vi "Part 2.vi"() -> ()   [LabVIEW 2020]
uses:
  <vilib>/Utility/file.llb/Read Delimited Spreadsheet (string).vi
panel:
  in  "Selection":enum16{"Name", "Country of Birth", "Age"}(ring)
  out "Histogram Graph":cluster{i32[], i32[]}(graph)
  out "sum":i32
  out "Array":string[](array[string])
  out "Map":map{string, i32}(c390)
  in  "Path":path
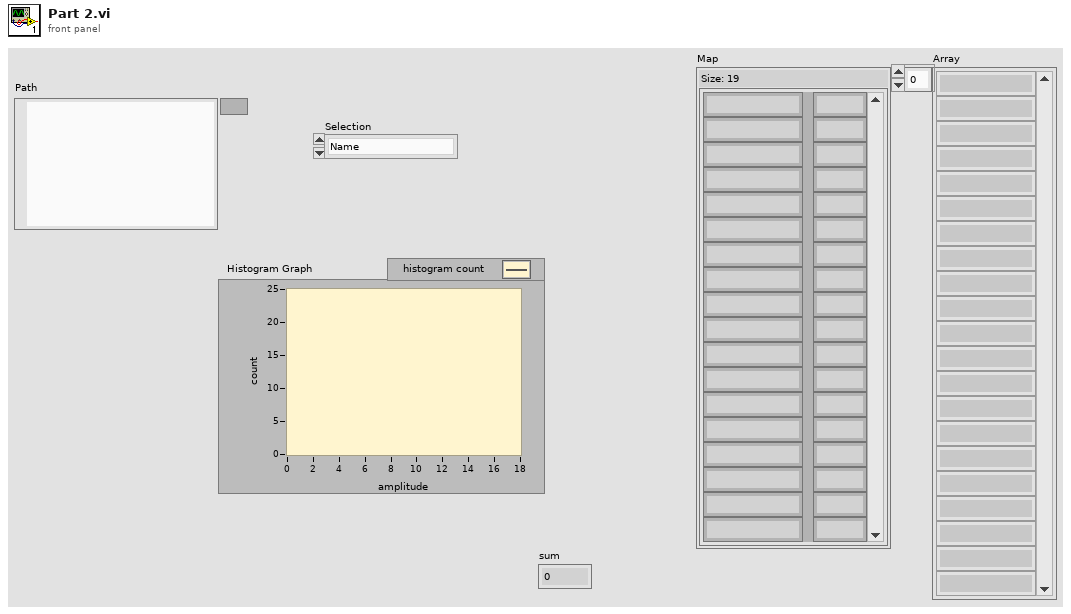
[diagram p1: front panel]
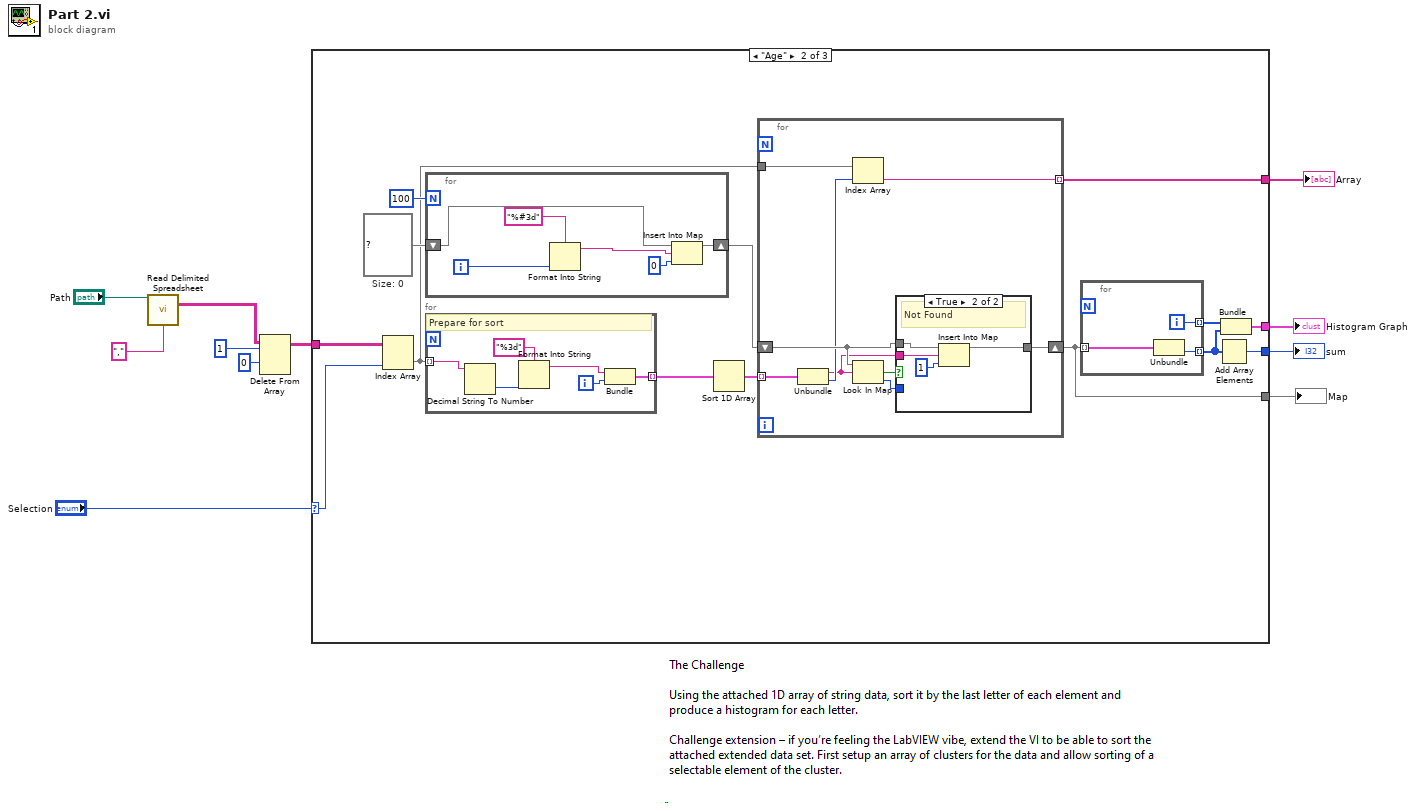
[diagram p0: block diagram]
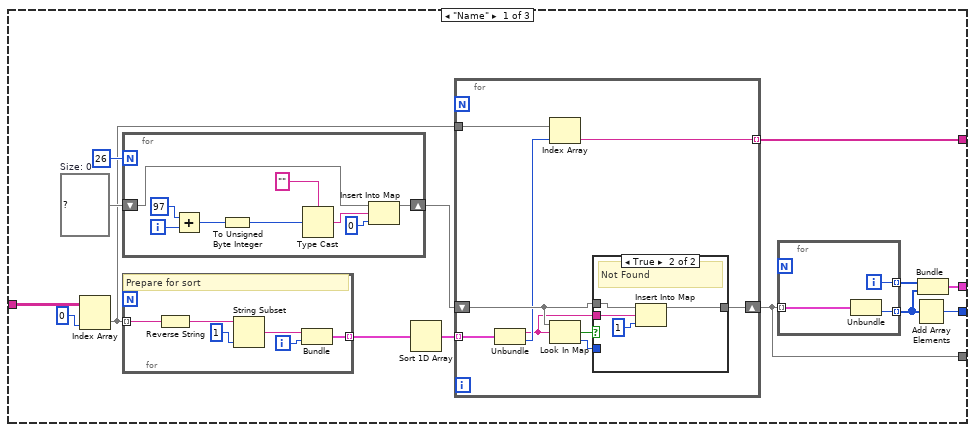
[diagram p2: hidden frame]
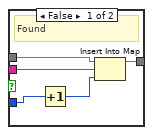
[diagram p3: hidden frame]
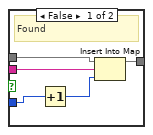
[diagram p4: hidden frame]
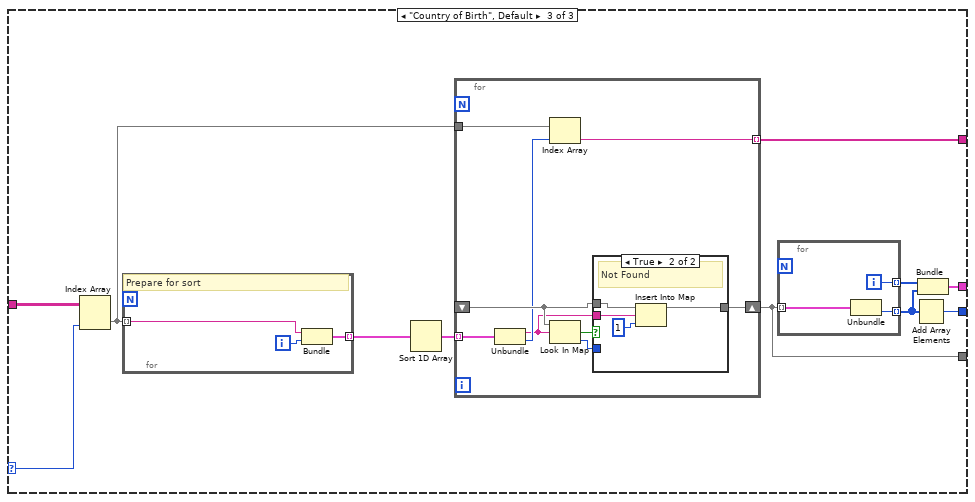
[diagram p5: hidden frame]
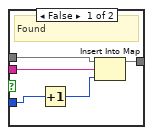
[diagram p6: hidden frame]
diagram:
  n1 = call-poly <vilib>:"Read Delimited Spreadsheet.vi"("file path (dialog if empty)"="Path", "delimiter (\\t)"="," ("delimiter (\\t)")) -> ("all rows"=w4:string[][])  [unwired: 8 in, 5 out]
  n2 = Delete From Array(array=w4, length=1, index (row)=0) -> (array with subset deleted=w3:string[][])  [unwired: 1 in, 1 out]
  n3 = case shown="\"Age\"" "Selection" {
    selector: "Selection" -> [_ w62 w109]
    tunnel: w3 -> [w25 w75 w119]
    tunnel: [w17 w68 w115] -> w9
    tunnel: [w16 w67 w114] -> w8
    tunnel: [w15 w66 w113] -> w7
    tunnel: [w14 w65 w112] -> w6
    frame "Name" {
      w22 = map{string, i32} {}  # Size: 0
      n4 = Index Array(array=w25, index (col)=0 ("disabled index (col)")) -> (element=w18:string[])  [unwired: 1 in]
      n5 = for {
        N: 26 -> [_]
        shift-right: [w50] -> w19
        shift-left: w22 -> [w51]
        i -> [w54]
        n6 = Add(x=97, y=w54) -> (x+y=w53:i32)
        n7 = To Unsigned Byte Integer(number=w53) -> (unsigned 8bit integer=w47:u8)
        n8 = Type Cast(type="", x=w47) -> (*(type *) &x=w49:string)
        n9 = Insert Into Map(map in=w51, key=w49, value=0) -> (map out=w50:map{string, i32})  [unwired: 2 out]
      }
      n10 = for {
        tunnel: w18 -> [w61] mode=indexing
        tunnel: [w56] -> w23 mode=indexing
        i -> [w57]
        # "Prepare for sort"
        n11 = Reverse String(1:w61) -> (0:w60:string)
        n12 = String Subset(string=w60, length (rest)=1 ("length (rest)")) -> (substring=w58:string)  [unwired: 1 in]
        n13 = Bundle(w58, w57) -> (w56:cluster{string, i32})  [unwired: 1 in]
      }
      n14 = Sort 1D Array(array=w23) -> (sorted array=w20:cluster{string, i32}[])
      n15 = for {
        tunnel: w20 -> [w37] mode=indexing
        shift-right: [w32] -> w16
        shift-left: w19 -> [w33]
        tunnel: w18 -> [w36]
        tunnel: [w35] -> w17 mode=indexing
        n16 = Unbundle(w37) -> (w30:string, w31:i32)
        n17 = Index Array(array=w36, index=w31) -> (element=w35:string)
        n18 = Look In Map(map=w33, key=w30) -> (key not found?=w34:bool, value=w29:i32)  [unwired: 1 in]
        n19 = case shown="True" w34 {
          tunnel: w33 -> [w42 w45]
          tunnel: [w41 w46] -> w32
          tunnel: w30 -> [w40 w44]
          tunnel: w29 -> [w39 _]
          frame False {
            # "Found"
            n20 = Increment(x=w39) -> (x+1=w38:i32)
            n21 = Insert Into Map(map in=w42, key=w40, value=w38) -> (map out=w41:map{string, i32})  [unwired: 2 out]
          }
          frame True {
            # "Not Found"
            n22 = Insert Into Map(map in=w45, key=w44, value=1) -> (map out=w46:map{string, i32})  [unwired: 2 out]
          }
        }
      }
      n23 = for {
        tunnel: w16 -> [w28] mode=indexing
        tunnel: [w27] -> w13 mode=indexing
        tunnel: [w26] -> w12 mode=indexing
        i -> [w26]
        n24 = Unbundle(w28) -> (w27:i32)  [unwired: 1 out]
      }
      n25 = Add Array Elements(numeric array=w13) -> (sum=w15:i32)
      n26 = Bundle(w12, w13) -> (w14:cluster{i32[], i32[]})  [unwired: 1 in]
    }
    frame "Age" {
      w73 = map{string, i32} {}  # Size: 0
      n27 = Index Array(array=w75, index (col)=w62) -> (element=w69:string[])  [unwired: 1 in]
      n28 = for {
        N: 100 -> [_]
        shift-right: [w101] -> w70
        shift-left: w73 -> [w102]
        i -> [w98]
        n29 = Format Into String(format string="%#3d", w98) -> (resulting string=w97:string)  [unwired: 2 in, 1 out]
        n30 = Insert Into Map(map in=w102, key=w97, value=0) -> (map out=w101:map{string, i32})  [unwired: 2 out]
      }
      n31 = for {
        tunnel: w69 -> [w104] mode=indexing
        tunnel: [w107] -> w74 mode=indexing
        i -> [w108]
        # "Prepare for sort"
        n32 = Decimal String To Number(string=w104) -> (number=w105:i32)  [unwired: 2 in, 1 out]
        n33 = Format Into String(format string="%3d", w105) -> (resulting string=w103:string)  [unwired: 2 in, 1 out]
        n34 = Bundle(w103, w108) -> (w107:cluster{string, i32})  [unwired: 1 in]
      }
      n35 = Sort 1D Array(array=w74) -> (sorted array=w71:cluster{string, i32}[])
      n36 = for {
        tunnel: w71 -> [w87] mode=indexing
        shift-right: [w82] -> w67
        shift-left: w70 -> [w83]
        tunnel: w69 -> [w86]
        tunnel: [w85] -> w68 mode=indexing
        n37 = Unbundle(w87) -> (w80:string, w81:i32)
        n38 = Index Array(array=w86, index=w81) -> (element=w85:string)
        n39 = Look In Map(map=w83, key=w80) -> (key not found?=w84:bool, value=w79:i32)  [unwired: 1 in]
        n40 = case shown="True" w84 {
          tunnel: w83 -> [w92 w95]
          tunnel: [w91 w96] -> w82
          tunnel: w80 -> [w90 w94]
          tunnel: w79 -> [w89 _]
          frame False {
            # "Found"
            n41 = Increment(x=w89) -> (x+1=w88:i32)
            n42 = Insert Into Map(map in=w92, key=w90, value=w88) -> (map out=w91:map{string, i32})  [unwired: 2 out]
          }
          frame True {
            # "Not Found"
            n43 = Insert Into Map(map in=w95, key=w94, value=1) -> (map out=w96:map{string, i32})  [unwired: 2 out]
          }
        }
      }
      n44 = for {
        tunnel: w67 -> [w78] mode=indexing
        tunnel: [w77] -> w64 mode=indexing
        tunnel: [w76] -> w63 mode=indexing
        i -> [w76]
        n45 = Unbundle(w78) -> (w77:i32)  [unwired: 1 out]
      }
      n46 = Add Array Elements(numeric array=w64) -> (sum=w66:i32)
      n47 = Bundle(w63, w64) -> (w65:cluster{i32[], i32[]})  [unwired: 1 in]
    }
    frame "Country of Birth", Default {
      n48 = Index Array(array=w119, index (col)=w109) -> (element=w116:string[])  [unwired: 1 in]
      n49 = for {
        tunnel: w116 -> [w141] mode=indexing
        tunnel: [w142] -> w118 mode=indexing
        i -> [w143]
        # "Prepare for sort"
        n50 = Bundle("String"=w141, w143) -> (w142:cluster{"String":string, i32})  [unwired: 1 in]
      }
      n51 = Sort 1D Array(array=w118) -> (sorted array=w117:cluster{"String":string, i32}[])
      n52 = for {
        tunnel: w117 -> [w131] mode=indexing
        shift-right: [w126] -> w114
        shift-left: _ -> [w127]
        tunnel: w116 -> [w130]
        tunnel: [w129] -> w115 mode=indexing
        n53 = Unbundle(w131) -> ("String"=w124:string, w125:i32)
        n54 = Index Array(array=w130, index=w125) -> (element=w129:string)
        n55 = Look In Map(map=w127, key=w124) -> (key not found?=w128:bool, value=w123:i32)  [unwired: 1 in]
        n56 = case shown="True" w128 {
          tunnel: w127 -> [w136 w139]
          tunnel: [w135 w140] -> w126
          tunnel: w124 -> [w134 w138]
          tunnel: w123 -> [w133 _]
          frame False {
            # "Found"
            n57 = Increment(x=w133) -> (x+1=w132:i32)
            n58 = Insert Into Map(map in=w136, key=w134, value=w132) -> (map out=w135:map{string, i32})  [unwired: 2 out]
          }
          frame True {
            # "Not Found"
            n59 = Insert Into Map(map in=w139, key=w138, value=1) -> (map out=w140:map{string, i32})  [unwired: 2 out]
          }
        }
      }
      n60 = for {
        tunnel: w114 -> [w122] mode=indexing
        tunnel: [w121] -> w111 mode=indexing
        tunnel: [w120] -> w110 mode=indexing
        i -> [w120]
        n61 = Unbundle(w122) -> ("value"=w121:i32)  [unwired: 1 out]
      }
      n62 = Add Array Elements(numeric array=w111) -> (sum=w113:i32)
      n63 = Bundle(w110, w111) -> (w112:cluster{i32[], i32[]})  [unwired: 1 in]
    }
  }
  "Map" <- w8
  "Array" <- w9
  "sum" <- w7
  "Histogram Graph" <- w6
